vi "AutoLoad.vi"(11 "Array":dbl[](array[numeric]) format="%0.3f") -> ()   [LabVIEW 2013]
uses:
  Rollers/Roller Control.ctl
  Rollers/Roller Mode.ctl
  Robot Global Data.vi
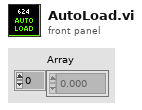
[diagram p1: front panel]
types:
  T1 = typedef "Roller Control.ctl" = cluster{"Mode":T2, "Front":enum16{"Stop", "Forward", "Reverse"}, "Back":enum16{"Stop", "Forward", "Reverse"}, "Reset":bool, "Front Piston":bool, "Halo":bool, "Net Piston":bool, "Carry Two":bool, "Hold":bool}
  T2 = typedef "Roller Mode.ctl" = enum16{"None", "Front", "Back", "Both", "Manual"}
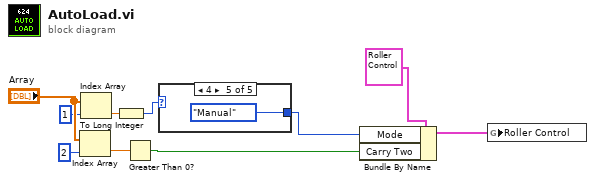
[diagram p0: block diagram]
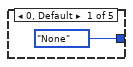
[diagram p2: hidden frame]
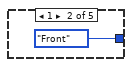
[diagram p3: hidden frame]
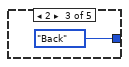
[diagram p4: hidden frame]
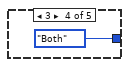
[diagram p5: hidden frame]
diagram:
  n1 = Index Array(array="Array", index=2) -> (element=w5:dbl)
  n2 = Index Array(array="Array", index=1) -> (element=w3:dbl)
  n3 = To Long Integer(number=w3) -> (32bit integer=w2:i32)
  n4 = Greater Than 0?(x=w5) -> (x > 0?=w4:bool)
  n5 = case shown="4" w2 {
    tunnel: [Roller_Mode."None" ("Mode") Roller_Mode."Front" ("Mode") Roller_Mode."Back" ("Mode") Roller_Mode."Both" ("Mode") Roller_Mode."Manual" ("Mode")] -> w1
    frame 0, Default {
    }
    frame 1 {
    }
    frame 2 {
    }
    frame 3 {
    }
    frame 4 {
    }
  }
  n6 = Bundle By Name(cluster=T1 {"Mode"=enum."None", "Front"=enum."Stop", "Back"=enum."Stop", "Reset"=FALSE, "Front Piston"=FALSE, "Halo"=FALSE, "Net Piston"=FALSE, "Carry Two"=FALSE, "Hold"=FALSE} ("Roller Control"), "Mode"=w1, "Carry Two"=w4) -> (w6:T1)
  n7 = global write "Robot Global Data.vi" "Roller Control"(w6) -> ()
